vi "Register (async) JSON.vi"(0 "WAMP Client in":refnum<class "WAMP Client.lvclass">, 1 "Options":string="{}", 5 "Procedure URI":string, 11 "error in (no error)":errorcluster) -> (4 "WAMP Client out":refnum<class "WAMP Client.lvclass">, 6 "notifier out":refnum<notifier>, 15 "error out":errorcluster)   [LabVIEW 2020, in "wamplv.lvlib" / "WAMP Client.lvclass"]
uses:
  WAMP Client.lvclass
  Private/Requests/Register/Register JSON/Register JSON.lvclass/Register JSON.ctl
  WAMP Client.lvclass/WAMP Client.ctl
  Private/Requests/Register/Register JSON/Register JSON.lvclass
  C:/local/wamplv/Private/Requests/IInternalMessage/IInternalMessage.lvclass
  C:/local/wamplv/Private/Requests/IGenericWithOutputInternalMessage/IGenericWithOutputInternalMessage/IGenericWithOutputInternalMessage.lvclass
  C:/local/wamplv/Private/Requests/Register/IRegister/IRegister.lvclass
  C:/local/wamplv/Private/Requests/IContainersNotiferOrEvents/IContainersNotiferOrEvents.lvclass
  C:/local/wamplv/Private/Requests/Register/Register JSON/Register JSON.lvclass
  Private/Message loop classes/ErrorOrSuccess JSON/ErrorOrSuccess JSON.lvclass
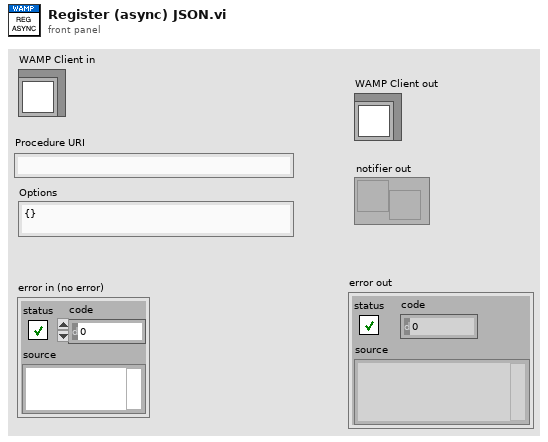
[diagram p1: front panel]
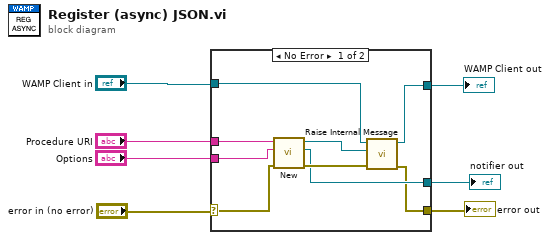
[diagram p0: block diagram]
diagram:
  n1 = case shown="No Error" "error in (no error)" {
    selector: "error in (no error)" -> [w10 w18]
    tunnel: [w8 w18] -> w6
    tunnel: [w15 w17] -> w4
    tunnel: "WAMP Client in" -> [w16 w17]
    tunnel: "Procedure URI" -> [w14 _]
    tunnel: "Options" -> [w13 _]
    tunnel: [w9 _] -> w1
    frame No Error {
      n2 = call "New.vi"("error in (no error)"=w10, "Options"=w13, "Procedure URI"=w14) -> ("error out"=w12:errorcluster, "notifier out"=w9:refnum<notifier>, "Register JSON out"=w11:refnum<class "Register JSON.lvclass">)  [unwired: 6 in]
      n3 = call "Raise Internal Message.vi"("error in (no error)"=w12, "IInternalMessage"=w11, "WAMP Client in"=w16) -> ("error out"=w8:errorcluster, "WAMP Client out"=w15:refnum<class "WAMP Client.lvclass">)  [unwired: 7 in]
    }
    frame Error {
    }
  }
  "error out" <- w6
  "WAMP Client out" <- w4
  "notifier out" <- w1
